vi "TW Update Project Internal Paths.vi"(7 "Rename Project":bool=TRUE, 8 "error in (no error)":errorcluster, 9 "Replace Subname":string="Template", 10 "New Subname":string, 11 "Project Path":path) -> (0 "error out":errorcluster)   [LabVIEW 2021, in "Plugin Generator.lvlib"]
uses:
  Plugin Generator.lvlib
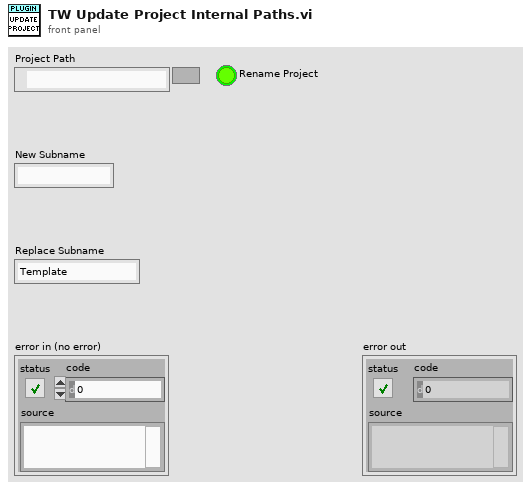
[diagram p1: front panel]
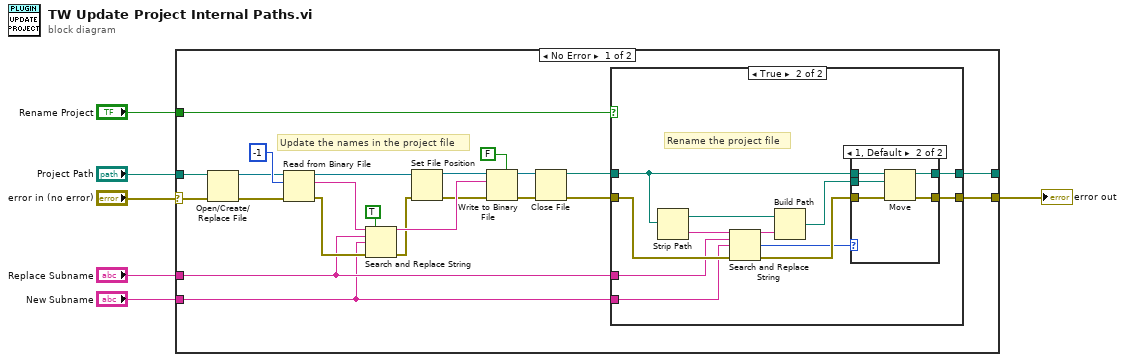
[diagram p0: block diagram]
diagram:
  n1 = case shown="No Error" "error in (no error)" {
    selector: "error in (no error)" -> [w13 w51]
    tunnel: [w18 w51] -> w1
    tunnel: [w17 _] -> _
    tunnel: "Project Path" -> [w12 _]
    tunnel: "New Subname" -> [w7 _]
    tunnel: "Replace Subname" -> [w8 _]
    tunnel: "Rename Project" -> [w9 _]
    frame No Error {
      # "Update the names in the project file"
      n2 = Open/Create/Replace File(file path (use dialog)=w12, error in=w13) -> (refnum out=w14:refnum<file>, error out=w16:errorcluster)  [unwired: 4 in, 1 out]
      n3 = Read from Binary File(8:w16, 10:-1 ("count (1)"), 11:w14) -> (0:w11:errorcluster, 2:w29:string, 3:w23:refnum<file>)  [unwired: 3 in, 1 out]
      n4 = Search and Replace String(replace all?=TRUE ("replace all? (F)"), input string=w29, search string=w8, replace string=w7, error in=w11) -> (result string=w26:string, error out=w10:errorcluster)  [unwired: 3 in, 2 out]
      n5 = Set File Position(refnum=w23, error in=w10) -> (refnum out=w22:refnum<file>, error out=w21:errorcluster)  [unwired: 2 in]
      n6 = Write to Binary File(file (use dialog)=w22, data=w26, error in=w21, 5:FALSE ("prepend array or string size? (T)")) -> (refnum out=w28:refnum<file>, error out=w27:errorcluster)  [unwired: 2 in, 1 out]
      n7 = Close File(refnum=w28, error in=w27) -> (path=w19:path, error out=w20:errorcluster)
      n8 = case shown="True" w9 {
        tunnel: w20 -> [w30 w38]
        tunnel: w19 -> [w31 w42]
        tunnel: [w30 w40] -> w18
        tunnel: [w31 w39] -> w17
        tunnel: w7 -> [_ w34]
        tunnel: w8 -> [_ w33]
        frame False {
        }
        frame True {
          # "Rename the project file"
          n9 = Strip Path(path=w42) -> (stripped path=w43:path, name=w36:string)
          n10 = Search and Replace String(input string=w36, search string=w33, replace string=w34, error in=w38) -> (result string=w35:string, number of replacements=w32:i32, error out=w37:errorcluster)  [unwired: 4 in, 1 out]
          n11 = Build Path(base path=w43, name or relative path=w35) -> (appended path=w41:path)
          n12 = case shown="1, Default" w32 {
            tunnel: w42 -> [w45 w50]
            tunnel: w41 -> [_ w49]
            tunnel: [w44 w48] -> w40
            tunnel: [w45 w47] -> w39
            tunnel: w37 -> [w44 w46]
            frame 0 {
            }
            frame 1, Default {
              n13 = Move(source path=w50, error in=w46, 10:w49) -> (error out=w48:errorcluster, 3:w47:path)  [unwired: 2 in, 1 out]
            }
          }
        }
      }
    }
    frame Error {
    }
  }
  "error out" <- w1
